vi "Builder.vi"(8 "error in (no error)":errorcluster) -> (0 "error out":errorcluster, 3 "Client out":refnum<class "Client.lvclass">)   [LabVIEW 2017, in "opcua.lvlib" / "Client.lvclass"]
uses:
  Client.lvclass
  Client.lvclass/Client.ctl
  opcua32.dll
  opcua.lvlib
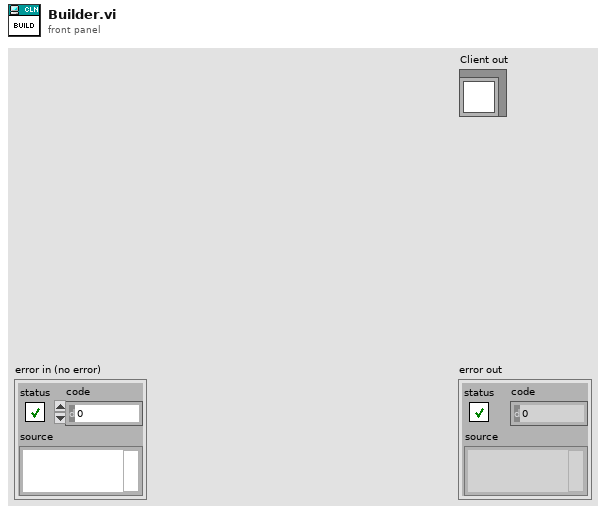
[diagram p1: front panel]
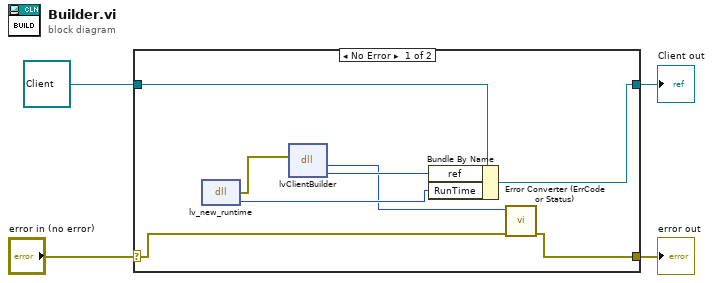
[diagram p0: block diagram]
diagram:
  n1 = case shown="No Error" "error in (no error)" {
    selector: "error in (no error)" -> [w7 w13]
    tunnel: [w6 w13] -> w3
    tunnel: [w11 w14] -> w1
    tunnel: refnum<class "Client.lvclass"> refnum ("Client in") -> [w12 w14]
    frame No Error {
      n2 = dll-call lib="C:/Users/Andrey/Desktop/opcua-labview/opcua-lvlib/opcua*.dll" fn="lv_new_runtime"() -> (error out=w8:errorcluster, "return type"=w9:u64)  [unwired: 3 in, 1 out]
      n3 = dll-call lib="C:/Users/Andrey/Desktop/opcua-labview/opcua-lvlib/opcua*.dll" fn="lvClientBuilder"(error in=w8) -> ("return type"=w5:i32, "client_ref"=w10:u64)  [unwired: 3 in, 2 out]
      n4 = Bundle By Name(cluster=w12, "ref"=w10, "RunTime"=w9) -> (w11:refnum<class "Client.lvclass">)
      n5 = call "Error Converter (ErrCode or Status).vi"("error in (no error)"=w7, "error code"=w5) -> ("error out"=w6:errorcluster)  [unwired: 9 in]
    }
    frame Error {
    }
  }
  "error out" <- w3
  "Client out" <- w1
